vi "Wiimote Read Button State.vi"(8 "error in (no error)":errorcluster, 9 "Wiimote Player #":i32=1, 11 "LV WiiMote Interface In":T2) -> (0 "error out":errorcluster, 2 "Wiimote Buttons":T1, 3 "LV WiiMote Interface out":T2)   [LabVIEW 2012, in "LV Wiimote Interface.lvclass"]
uses:
  LV Wiimote Interface.lvclass
  Controls/LV Wiimote Interface.ctl
  Controls/Wiimote Buttons.ctl
  C:/Program Files/National Instruments/LabVIEW 2012/vi.lib/LabVIEW Hacker/WiiMote/Dependencies/WiimoteLib.dll
  Program Files/National Instruments/LabVIEW 2012/vi.lib/LabVIEW Hacker/WiiMote/Dependencies/WiimoteLib.dll
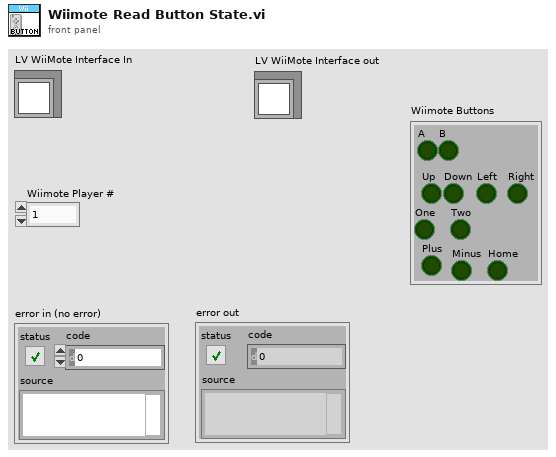
[diagram p1: front panel]
types:
  T1 = typedef "LV Wiimote Interface.lvclass/Wiimote Buttons.ctl" = cluster{"A":bool, "B":bool, "Up":bool, "Down":bool, "Left":bool, "Right":bool, "One":bool, "Two":bool, "Plus":bool, "Minus":bool, "Home":bool}
  T2 = typedef "LV Wiimote Interface.ctl" = refnum<class "LV Wiimote Interface.lvclass">
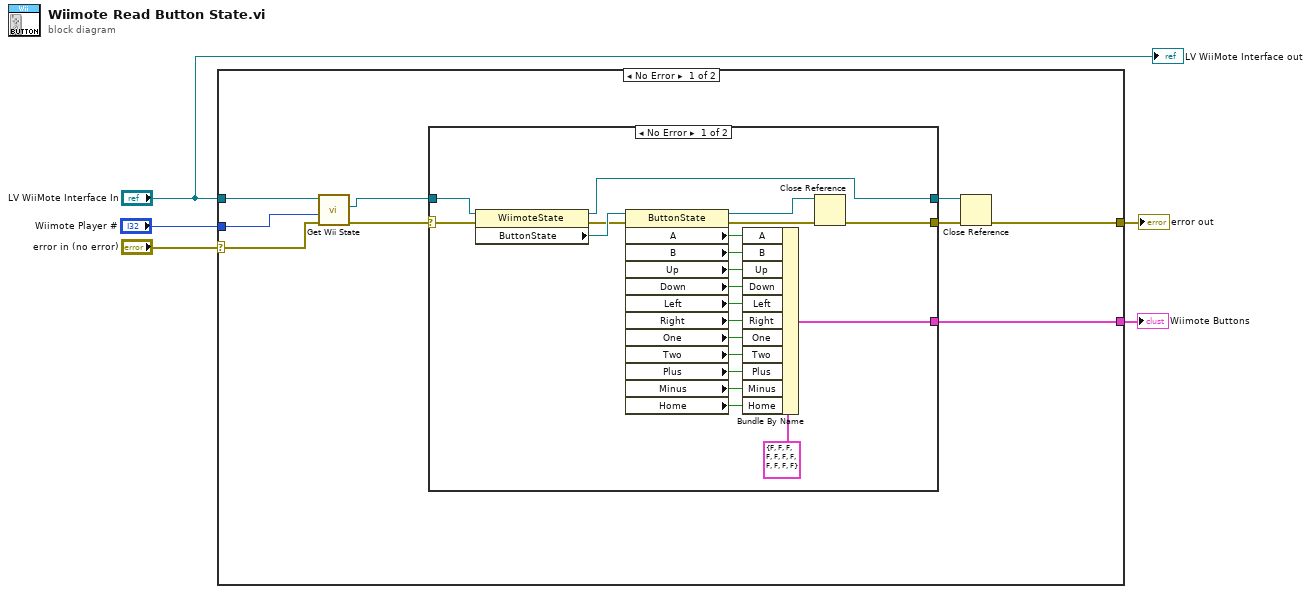
[diagram p0: block diagram]
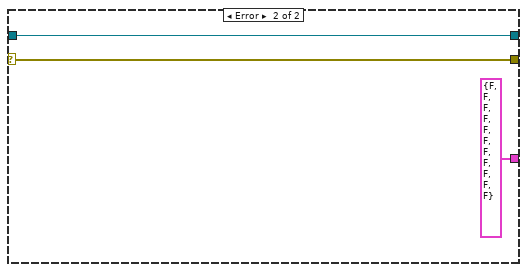
[diagram p2: hidden frame]
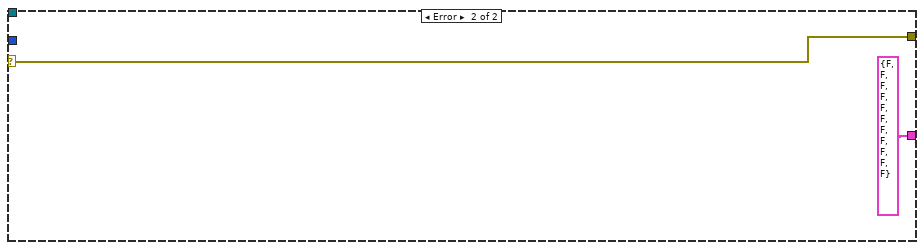
[diagram p3: hidden frame]
diagram:
  n1 = case shown="No Error" "error in (no error)" {
    selector: "error in (no error)" -> [w12 w40]
    tunnel: "LV WiiMote Interface In" -> [w14 _]
    tunnel: "Wiimote Player #" -> [w7 _]
    tunnel: [w13 T1 {"A"=FALSE, "B"=FALSE, "Up"=FALSE, "Down"=FALSE, "Left"=FALSE, "Right"=FALSE, "One"=FALSE, "Two"=FALSE, "Plus"=FALSE, "Minus"=FALSE, "Home"=FALSE} ("Wiimote Buttons")] -> w3
    tunnel: [w8 w40] -> w1
    frame No Error {
      n2 = call "Get Wii State.vi"("error in (no error)"=w12, "Wiimote Player #"=w7, "LV Wiimote Interface in"=w14) -> ("error out"=w11:errorcluster, "WiimoteState"=w6:refnum<k24>)  [unwired: 6 in, 1 out]
      n3 = case shown="No Error" w11 {
        selector: w11 -> [w17 w38]
        tunnel: w6 -> [w35 w36]
        tunnel: [w20 T1 {"A"=FALSE, "B"=FALSE, "Up"=FALSE, "Down"=FALSE, "Left"=FALSE, "Right"=FALSE, "One"=FALSE, "Two"=FALSE, "Plus"=FALSE, "Minus"=FALSE, "Home"=FALSE} ("Wiimote Buttons")] -> w13
        tunnel: [w16 w38] -> w10
        tunnel: [w15 w36] -> w9
        frame No Error {
          n4 = property class="WiimoteState"(reference=w35, error in=w17) -> (reference out=w15:refnum<k24>, error out=w33:errorcluster, "ButtonState"=w34:refnum<k24>)
          n5 = property class="ButtonState"(reference=w34, error in=w33) -> (reference out=w18:refnum<k24>, error out=w19:errorcluster, "A"=w31:bool, "B"=w30:bool, "Up"=w29:bool, "Down"=w28:bool, "Left"=w27:bool, "Right"=w26:bool, "One"=w25:bool, "Two"=w24:bool, "Plus"=w23:bool, "Minus"=w22:bool, "Home"=w21:bool)
          n6 = Bundle By Name(cluster=T1 {"A"=FALSE, "B"=FALSE, "Up"=FALSE, "Down"=FALSE, "Left"=FALSE, "Right"=FALSE, "One"=FALSE, "Two"=FALSE, "Plus"=FALSE, "Minus"=FALSE, "Home"=FALSE} ("Wiimote Buttons"), "A"=w31, "B"=w30, "Up"=w29, "Down"=w28, "Left"=w27, "Right"=w26, "One"=w25, "Two"=w24, "Plus"=w23, "Minus"=w22, "Home"=w21) -> (w20:T1)
          n7 = Close Reference(reference=w18, error in (no error)=w19) -> (error out=w16:errorcluster)
        }
        frame Error {
        }
      }
      n8 = Close Reference(reference=w9, error in (no error)=w10) -> (error out=w8:errorcluster)
    }
    frame Error {
    }
  }
  "error out" <- w1
  "Wiimote Buttons" <- w3
  "LV WiiMote Interface out" <- "LV WiiMote Interface In"
